vi "teststatic.vi"(11 "GIC Input":T2={"     Use ?\nOff       On"=[FALSE, TRUE, FALSE, TRUE], "Mode:"=FALSE, "Extra Port"="", "Hokuyo Port"="COM7", "Tx Prop  Port"="COM6", "Compass Port"="", "GPS Port"="", "Num of WPs"=0, "WP Lats and Longs"={"WP Lats"=[], "WP Longs"=[]}, "Obst Lats and Longs"={"Obst Lats"=[], "Obst Longs"=[]}, "Parameters"=[], "GPS Data"=[], "Compass"=0.0, "LMS Vector"=[], "Vision Vector"=[], "Direction Cmd"=0.0, "Speed Cmd"=0.0, "WP Vector"=[], "WP Number"=0, "Extra"=0, "SW Map"=[], "Path Cluster"={"Path x node"=[], "Path y node"=[]}, "Sim Course"=[]} {"Obst Lats and Longs"."Obst Longs" format="%#_8g"; "Obst Lats and Longs"."Obst Lats" format="%#_8g"}) -> (3 "GIC Output":T1={"     Use ?\nOff       On"=[FALSE, TRUE, FALSE, TRUE], "Mode:"=FALSE, "Extra Port"="", "Hokuyo Port"="COM7", "Tx Prop Port"="COM6", "Compass Port"="", "GPS Port"="", "Num of WPs"=0, "WP Lats and Longs"={"WP Lats"=[], "WP Longs"=[]}, "Obst Lats and Longs"={"Obst Lats"=[], "Obst Longs"=[]}, "Parameters"=[], "GPS Data"=[], "Compass"=0.0, "LMS Vector"=[], "Vision Vector"=[], "Direction Cmd"=0.0, "Speed Cmd"=0.0, "WP Vector"=[], "WP Number"=0, "Extra"=0, "SW Map"=[], "Path Cluster"={"Path x node"=[], "Path y node"=[]}, "Sim Course"=[]} {"Obst Lats and Longs"."Obst Longs" format="%#_8g"; "Obst Lats and Longs"."Obst Lats" format="%#_8g"})   [LabVIEW 2014]
panel:
  in  "WPs":dbl[](array[numeric])=[0.0, 0.0, 0.0, 0.0, 0.0, 0.0, 0.0, 0.0, 0.0, 0.0]
  # "teststatic"
  # "Input:"
  # "Output"
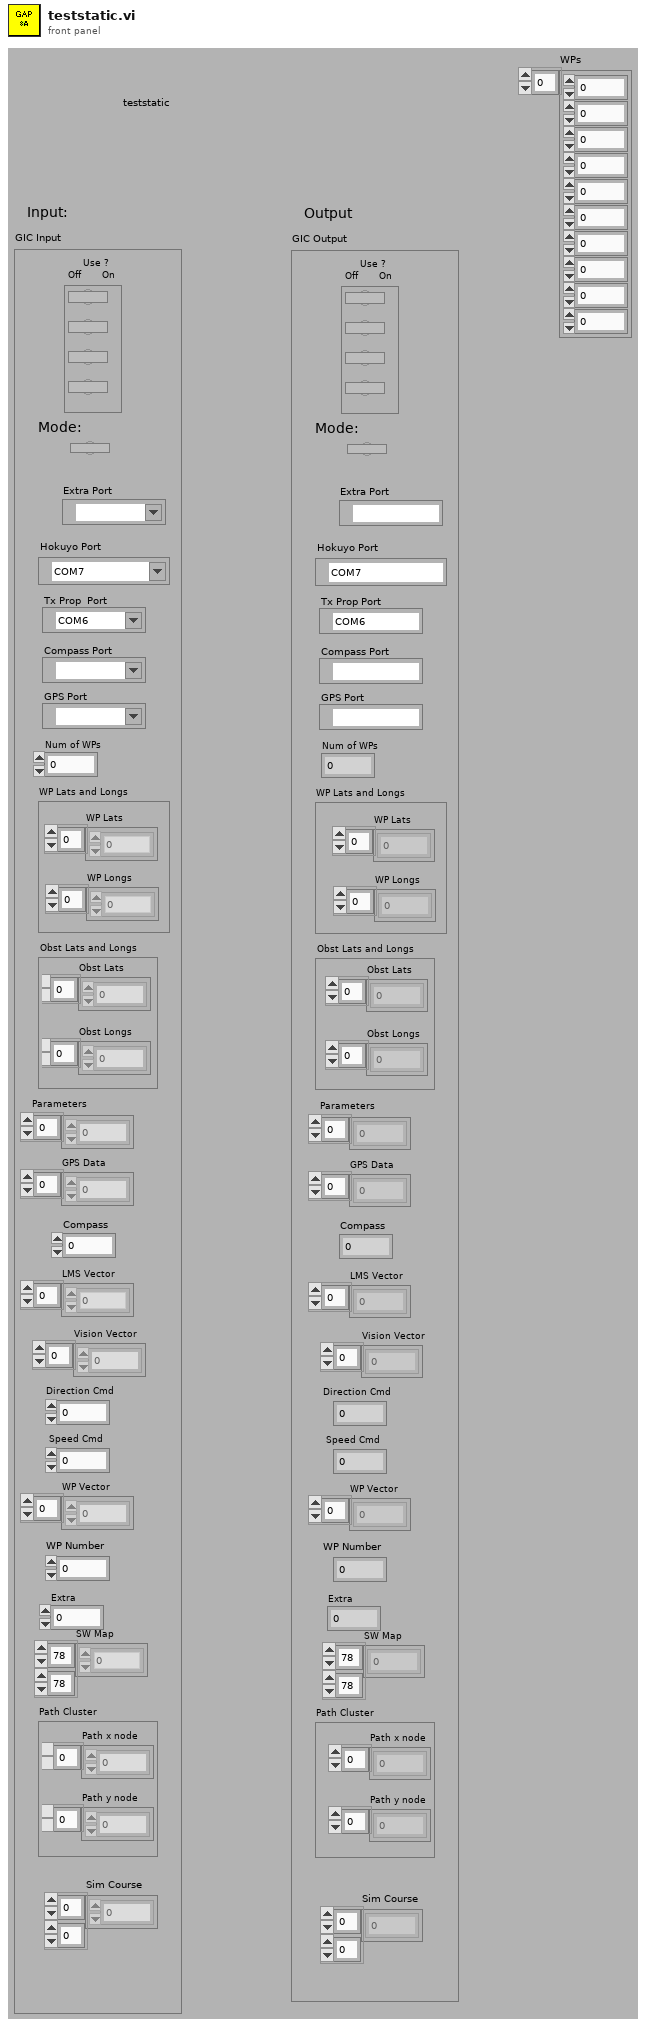
[diagram p1: front panel]
types:
  T1 = cluster{"     Use ?\nOff       On":bool[], "Mode:":bool, "Extra Port":refnum<visa-resource-name>, "Hokuyo Port":refnum<visa-resource-name>, "Tx Prop Port":refnum<visa-resource-name>, "Compass Port":refnum<visa-resource-name>, "GPS Port":refnum<visa-resource-name>, "Num of WPs":i16, "WP Lats and Longs":cluster{"WP Lats":dbl[], "WP Longs":dbl[]}, "Obst Lats and Longs":cluster{"Obst Lats":dbl[], "Obst Longs":dbl[]}, "Parameters":dbl[], "GPS Data":dbl[], "Compass":dbl, "LMS Vector":dbl[], "Vision Vector":dbl[], "Direction Cmd":dbl, "Speed Cmd":dbl, "WP Vector":dbl[], "WP Number":i32, "Extra":i16, "SW Map":i32[][], "Path Cluster":cluster{"Path x node":dbl[], "Path y node":dbl[]}, "Sim Course":i8[][]}
  T2 = cluster{"     Use ?\nOff       On":bool[], "Mode:":bool, "Extra Port":refnum<visa-resource-name>, "Hokuyo Port":refnum<visa-resource-name>, "Tx Prop  Port":refnum<visa-resource-name>, "Compass Port":refnum<visa-resource-name>, "GPS Port":refnum<visa-resource-name>, "Num of WPs":i16, "WP Lats and Longs":cluster{"WP Lats":dbl[], "WP Longs":dbl[]}, "Obst Lats and Longs":cluster{"Obst Lats":dbl[], "Obst Longs":dbl[]}, "Parameters":dbl[], "GPS Data":dbl[], "Compass":dbl, "LMS Vector":dbl[], "Vision Vector":dbl[], "Direction Cmd":dbl, "Speed Cmd":dbl, "WP Vector":dbl[], "WP Number":i32, "Extra":i16, "SW Map":i32[][], "Path Cluster":cluster{"Path x node":dbl[], "Path y node":dbl[]}, "Sim Course":i8[][]}
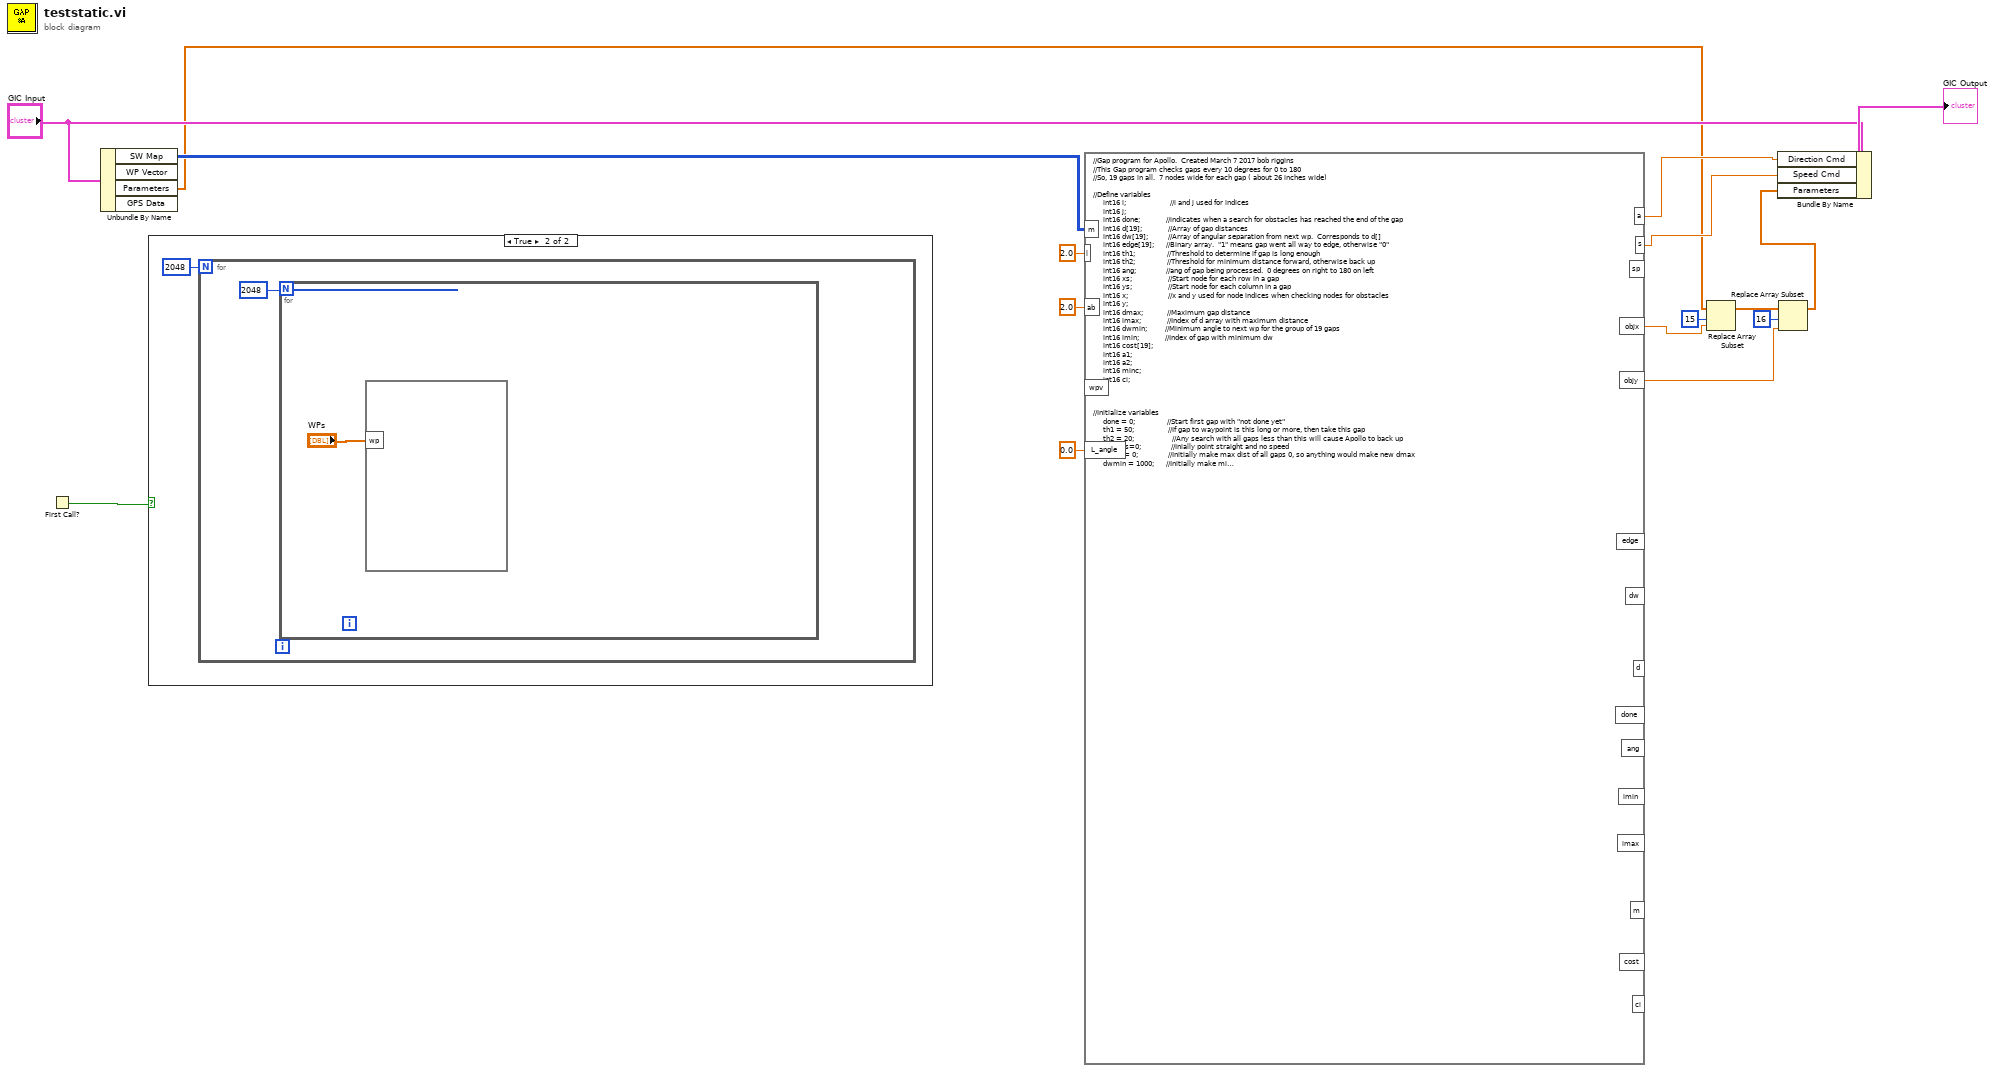
[diagram p0: block diagram]
diagram:
  n1 = First Call?() -> (First Call?: T/F=w7:bool)
  n2 = Unbundle By Name("GIC Input") -> ("SW Map"=w5:i32[][], "Parameters"=w1:dbl[])  [unwired: 2 out]
  n3 = case shown="True" w7 {
    frame False {
    }
    frame True {
      n4 = for {
        N: 2048 -> [_]
        n5 = for {
          N: 2048 -> [_]
          n6 = formula code=""("wp"="WPs") -> ()
        }
      }
    }
  }
  n7 = formula code="//Gap program for Apollo.  Created March 7 2017 bob riggins\n//This Gap program checks gaps every 10 degrees for 0 to 180\n//So, 19 gaps in all.  7 nodes wide for each gap ( about 26 inches wide)\n\n//Define variables\n     int16 i;                      //i and j used for indices\n     int16 j;\n     int16 done;             //indicates when a search for obstacles has reached the end of the gap\n     int16 d[19];             //Array of gap distances\n     int16 dw[19];          //Array of angular separation from next wp.  Corresponds to d[]\n     int16 edge[19];      //Binary array.  \"1\" means gap went all way to edge, otherwise \"0\"\n     int16 th1;                //Threshold to determine if gap is long enough\n     int16 th2;                //Threshold for minimum distance forward, otherwise back up\n     int16 ang;               //ang of gap being processed.  0 degrees on right to 180 on left\n     int16 xs;                  //Start node for each row in a gap\n     int16 ys;                  //Start node for each column in a gap\n     int16 x;                    //x and y used for node indices when checking nodes for obstacles\n     int16 y;\n     int16 dmax;            //Maximum gap distance\n     int16 imax;             //Index of d array with maximum distance\n     int16 dwmin;         //Minimum angle to next wp for the group of 19 gaps\n     int16 imin;             //Index of gap with minimum dw\n     int16 cost[19];\n     int16 a1;\n     int16 a2;\n     int16 minc;\n     int16 ci;\n     \n     \n\n//Initialize variables\n     done = 0;                //Start first gap with \"not done yet\"\n     th1 = 50;                 //If gap to waypoint is this long or more, then take this gap\n     th2 = 20;                   //Any search with all gaps less than this will cause Apollo to back up\n     a=90; s=0;               //Inially point straight and no speed\n     dmax = 0;               //Initially make max dist of all gaps 0, so anything would make new dmax\n     dwmin = 1000;      //Initially make min dw ridiculously high so any gap angle is beterr for start\n                                     //Find dw[i],  angular separations from wp angle, and best index with min\n     for(i = 0; i < 19; i = i + 1)\n          {\n               dw[i] = abs(wpv[0] + (10 * i) - 90);\n               if(dw[i] < dwmin) {dwmin = dw[i]; imin = i;}\n          } \n     minc = 10000;\n     a1 = 2;\n     a2 = 1;\n\n//Find d[5].....d[9] for angles 50 to 90\n     for(i = 0; i < 5; i = i + 1)\n          {\n               ang = (50 + (10 * i));\n               y = 60; xs = 37;\n               done = 0;\n               while (done  == 0)\n                    {\n                         if(y < 0 || xs+ 7 > 79)  {done = 1; edge[i + 5] = 1;}\n                         for(j = 0;j < 7;j = j + 1)\n                              { if(m[y][xs + j] > 1200)  {done = 1;}}\n                         if(done == 0)\n                              {\n                                   d[i + 5] = d[i + 5] + 1; y = y - 1;\n                                   xs = int((60 - y) * tan((90 - ang)*pi/180) + .5) + 37;\n                              }\n                    }\n                if(d[i + 5] > dmax)  {dmax = d[i + 5]; imax = i + 5;}    \n          }      \n\n//Find d[10].....d[13] for angles 100 to 1300\n     for(i = 0; i < 4; i = i + 1)\n          {\n               ang = (100 + (10 * i));\n               y = 60; xs = 43;\n               done = 0;\n               while (done  == 0)\n                    {\n                         if(y < 0 || xs - 7 < 0)  {done = 1; edge[i + 10] = 1;}\n                         for(j = 0;j < 7;j = j + 1)\n                              { if(m[y][xs - j] > 1200)  {done = 1;}}\n                         if(done == 0)\n                              {\n                                   d[i + 10] = d[i + 10] + 1; y = y - 1;\n                                   xs = 43 - int((60 - y) * tan((ang - 90)*pi/180) + .5);\n                              }\n                    }\n                if(d[i + 10] > dmax)  {dmax = d[i + 10]; imax = i + 10;}\n          }      \n\n//Find d[0].....d[4] for angles 0 to 40\n     for(i = 0; i < 5; i = i + 1)\n          {\n               ang = (10 * i);\n               x = 40; ys = 63;\n               done = 0;\n               while (done  == 0)\n                    {\n                         if(x > 79)  {done = 1; edge[i] = 1;}\n                         for(j = 0;j < 7;j = j + 1)\n                              { if(m[ys - j][x] > 1200)  {done = 1;}}\n                         if(done == 0)\n                              {\n                                   d[i] = d[i] + 1; x = x + 1;\n                                   ys = 63 - int((x - 40) * tan((ang)*pi/180) + .5);\n                              }\n                    }\n                if(d[i] > dmax)  {dmax = d[i]; imax = i;}\n          }\n\n//Find d[14].....d[18] for angles 140 to 180\n     for(i = 0; i < 5; i = i + 1)\n          {\n               ang = 140 + (10 * i);\n               x = 40; ys = 63;\n               done = 0;\n               while (done  == 0)\n                    {\n                         if(x < 0)  {done = 1; edge[i + 14] = 1;}\n                         for(j = 0; j < 7; j = j + 1)\n                              { if(m[ys - j][x] > 1200)  {done = 1;}}\n                         if(done == 0)\n                              {\n                                   d[i + 14] = d[i + 14] + 1; x = x - 1;\n                                   ys = 63 - int((40 - x) * tan((180 - ang)*pi/180) + .5);\n                              }\n                    }\n                if(d[i + 14] > dmax)  {dmax = d[i + 14]; imax = i + 14;}\n          }      \n\n//If WP dist is less than a rectangle dist that is closest in angle to wp, go that way\n//Or if rect angle that is closest to wp has dist at least th1, go that way\n//Reset done variable and use it to indicate if have an \"s\" and an \"a\"\n     done = 0;\n     if( d[imin] >= wpv[1] * 10 || d[imin] > th1)     \n          {s = d[imin]; a = imin *10; done = 1;}\n     if(edge[imin] ==1)  \n           {s = d[imin]; a = imin *10; done = 1;}\n\n//If done then set objx and objy\n      if (done ==1)\n          {\n               objx=40+cos(a*0.017453)*s;\n               objy=60-sin(a*0.017453)*s;\n          }\n\n//Next set up weighted parameter array combining cost of distance and closeness to wp\n     if(done == 0)\n          {\n               for(i = 0; i < 19; i = i + 1)\n                    {\n                         cost[i] = a1 * 4 * (62 - d[i])+a2 * dw[i];\n                         if (cost[i] < minc) {minc = cost[i]; ci = i;}\n                    } \n               if(d[ci] > th2)\n                    {\n                         //a = ci * 10; s = d[ci]; done = 1;\n                         if(ci < 18 && ci > 0)\n                              {\n                                   a = ci * 10 + int((5 * (d[ci + 1] - d[ci - 1])) / 62 + .5);\n                              }\n                         else\n                              {a = ci * 10;}         \n                         s = d[ci]; done = 1;\n                         objx=40+cos(a*0.017453)*s;\n                         objy=60-sin(a*0.017453)*s;\n                    }\n               else\n                    {s=30;a=270; objx=40; objy = 79;}\n          }\n\n\n//Make speed command only the verticle component for sabertooth mixed mode\n     sp = (71* abs(objy - 60))/60;"("m"=w5, "l"=2.0 ("input variable"), "ab"=2.0 ("input variable"), "L_angle"=0.0 ("input variable")) -> ("a"=w10:dbl, "s"=w8:dbl, "objx"=w12:dbl, "objy"=w11:dbl)  [unwired: 1 in, 11 out]
  n8 = Replace Array Subset(array=w1, new element=w12, index=15) -> (w15:dbl[])
  n9 = Replace Array Subset(array=w15, new element=w11, index=16) -> (w13:dbl[])
  n10 = Bundle By Name(cluster="GIC Input", "Direction Cmd"=w10, "Speed Cmd"=w8, "Parameters"=w13) -> (→"GIC Output":T2)
